vi "LoadRefs.vi"(3 "error in":errorcluster) -> (8 "Références à enregistrer":dbl[][](array[numeric]), 10 "error out":errorcluster)   [LabVIEW 2013]
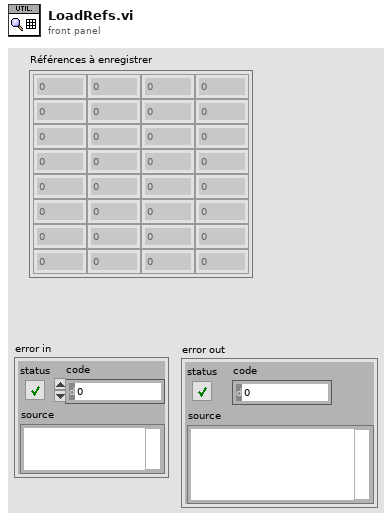
[diagram p1: front panel]
types:
  T1 = enum16{"open", "replace", "create", "open or create", "replace or create", "replace or create with confirmation"}
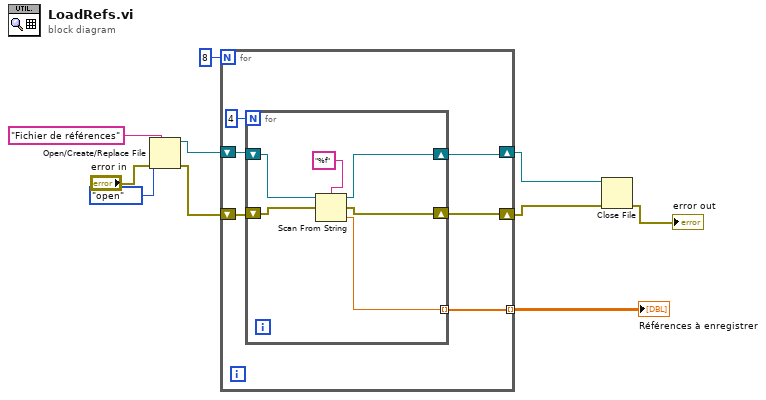
[diagram p0: block diagram]
diagram:
  n1 = Open/Create/Replace File(error in="error in", prompt="Fichier de références", operation (0:open)=T1."open") -> (refnum out=w4:refnum<file>, error out=w6:errorcluster)  [unwired: 3 in, 1 out]
  n2 = for {
    N: 8 -> [_]
    shift-right: [w11] -> w2
    shift-left: w6 -> [w15]
    tunnel: [w14] -> w5 mode=indexing
    shift-right: [w12] -> w3
    shift-left: w4 -> [w13]
    n3 = for {
      N: 4 -> [_]
      shift-right: [w20] -> w11
      shift-left: w15 -> [w21]
      shift-right: [w17] -> w12
      shift-left: w13 -> [w18]
      tunnel: [w19] -> w14 mode=indexing
      n4 = Scan From String("%f" ("format string"), w18, w21) -> (w17:refnum<file>, w20:errorcluster, output 1=w19:dbl)  [unwired: 1 in]
    }
  }
  "Références à enregistrer" <- w5
  n5 = Close File(refnum=w3, error in=w2) -> (error out=→"error out":errorcluster)  [unwired: 1 out]
